vi "main.vi"() -> ()   [LabVIEW 2012]
uses:
  SensorSettingCtl.ctl
  SensorTypes.ctl
  states.ctl
  globalVariables.vi
panel:
  in  "cancel button":bool
  out "TestLED":bool
  in  "Path for measuring results":path
  in  "Configuration of sensors":T1[](array[typedef])=[{"Sensor type"=enum."please select sensor", "Sensor on"=FALSE, "VISA resource name"="", "current transfer ratio"=0.0, "DMM Channel"="", "NPLC"=2, "Range"=enum."Maximum"}, {"Sensor type"=enum."ITL 900 (Analogue)", "Sensor on"=TRUE, "VISA resource name"="", "current transfer ratio"=0.0, "DMM Channel"="", "NPLC"=2, "Range"=enum."Maximum"}, {"Sensor type"=enum."CAB 300-C SP3 (CAN)", "Sensor on"=TRUE, "VISA resource name"="", "current transfer ratio"=0.0, "DMM Channel"="", "NPLC"=2, "Range"=enum."Maximum"}] {"NPLC" items=[".02", ".2", "1", "2", "10", "20", "100", "200", "Minimum", "Maximum"]}
  in  "start Button":bool
  out "Error Flag":bool
  # "Measurement of Current Sensors from LEM"
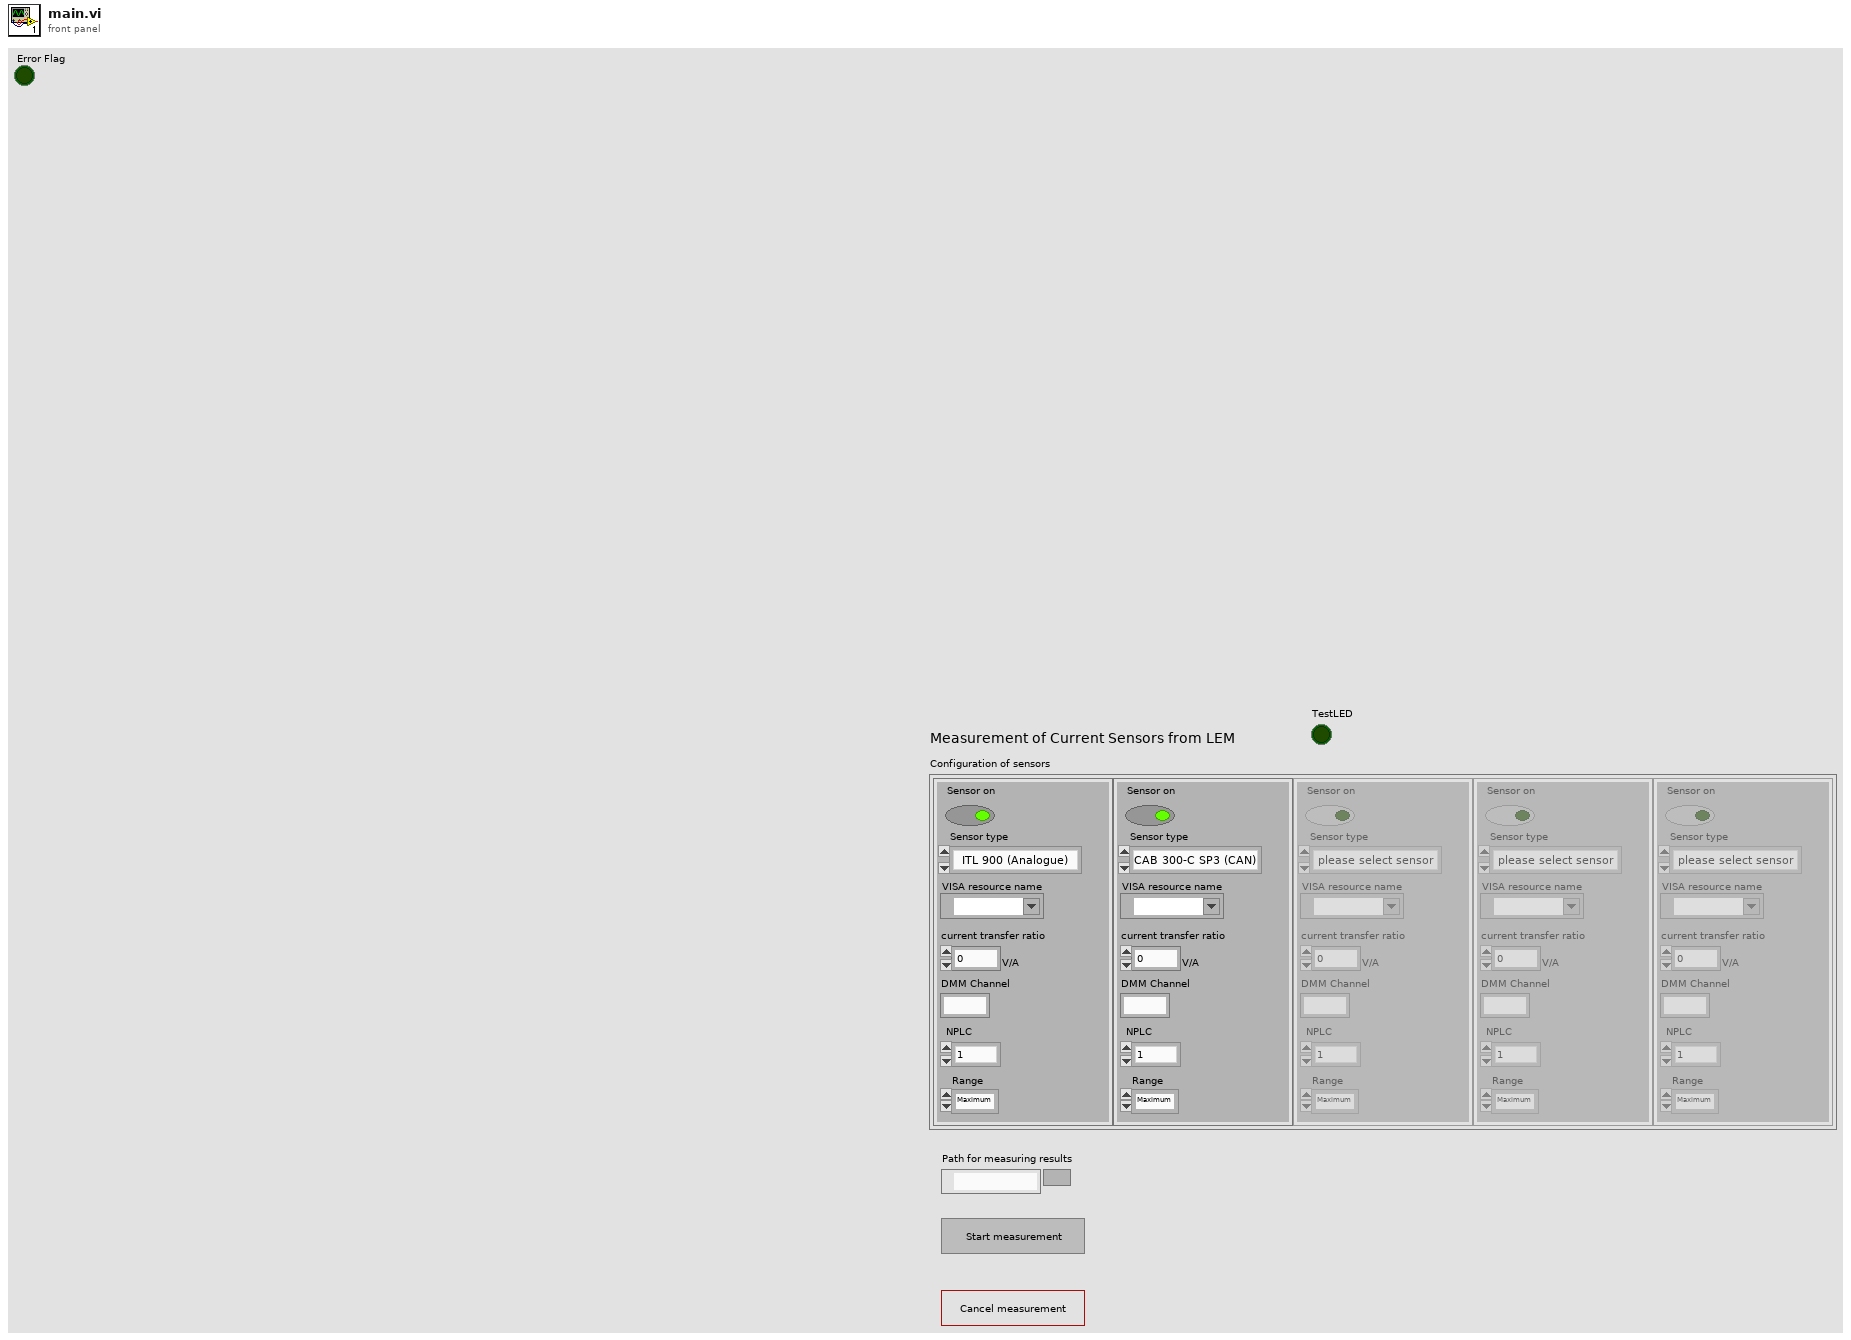
[diagram p1: front panel]
types:
  T1 = typedef "SensorSettingCtl.ctl" = cluster{"Sensor type":T2, "Sensor on":bool, "VISA resource name":refnum<visa-resource-name>, "current transfer ratio":dbl[unit], "DMM Channel":string, "NPLC":u16, "Range":enum16{"100 mV", "1 V", "10 V", "100 V", "300 V", "Minimum", "Maximum"}}
  T2 = typedef "SensorTypes.ctl" = enum16{"please select sensor", "ITL 900 (Analogue)", "CAB 300-C SP3 (CAN)", "xyz TODO (LIN)", "xyz TODO (Analogue)", "xyz TODO (CAN)"}
  T3 = typedef "states.ctl" = enum16{"init", "wait for user confirm", "start sensors", "measure", "terminate"}
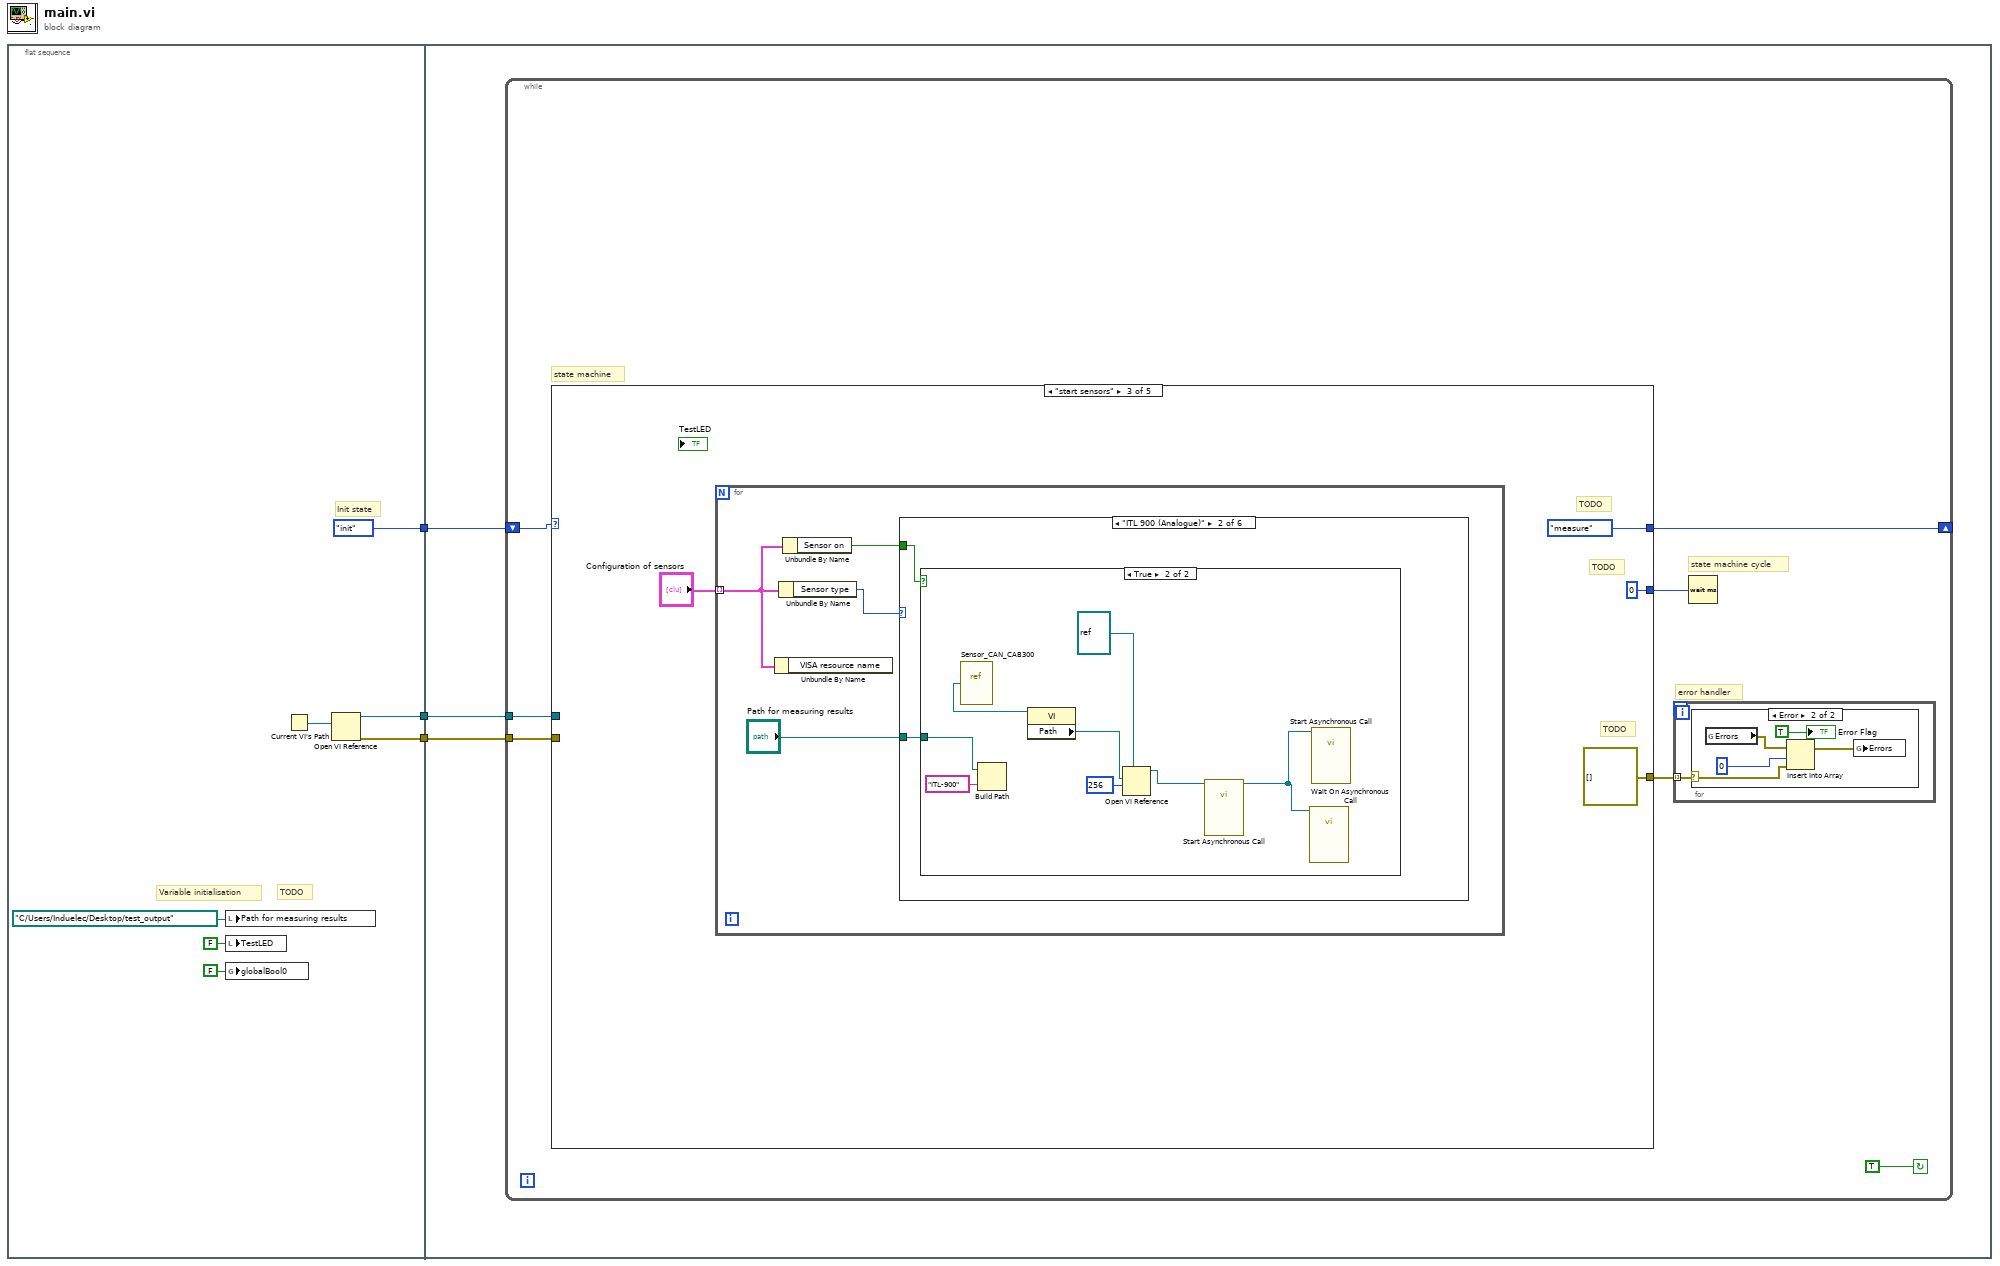
[diagram p0: block diagram]
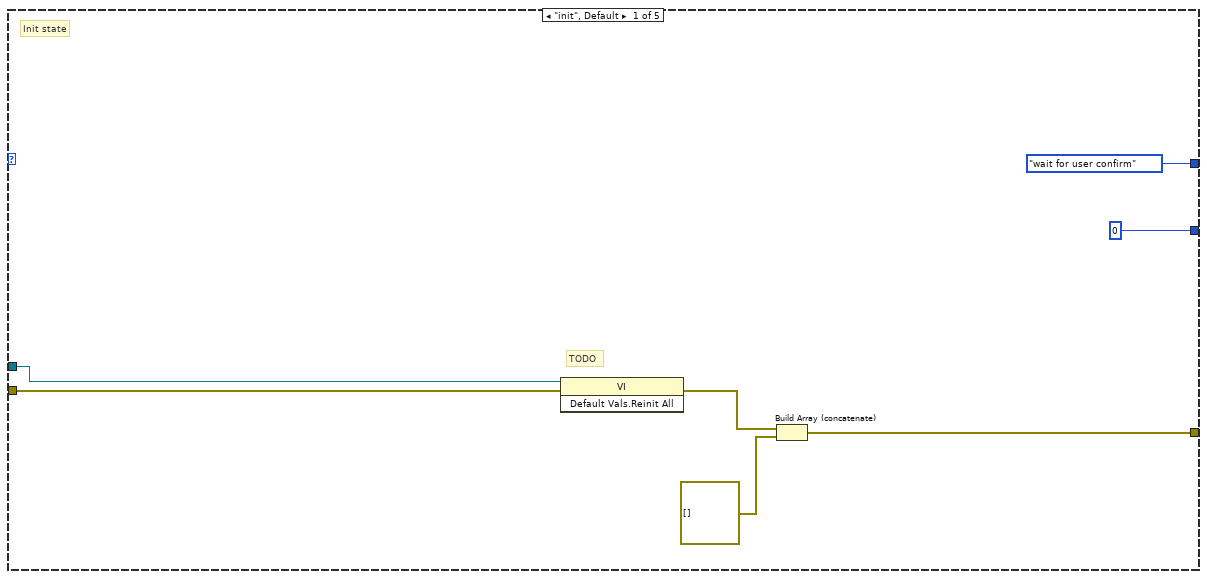
[diagram p3: hidden frame]
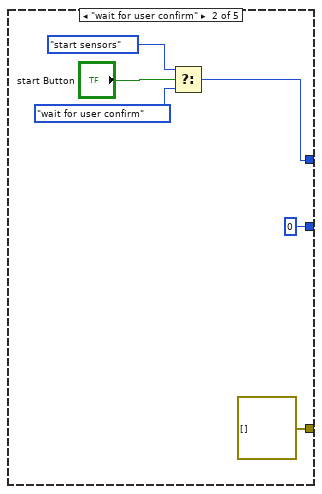
[diagram p4: hidden frame]
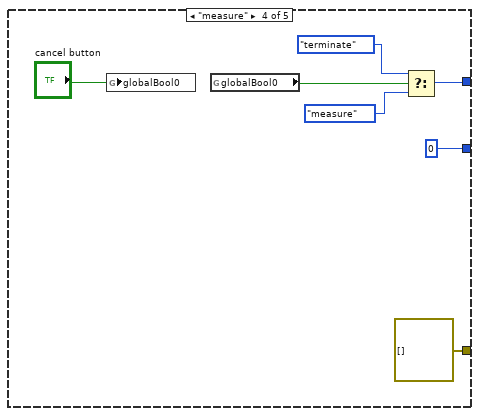
[diagram p11: hidden frame]
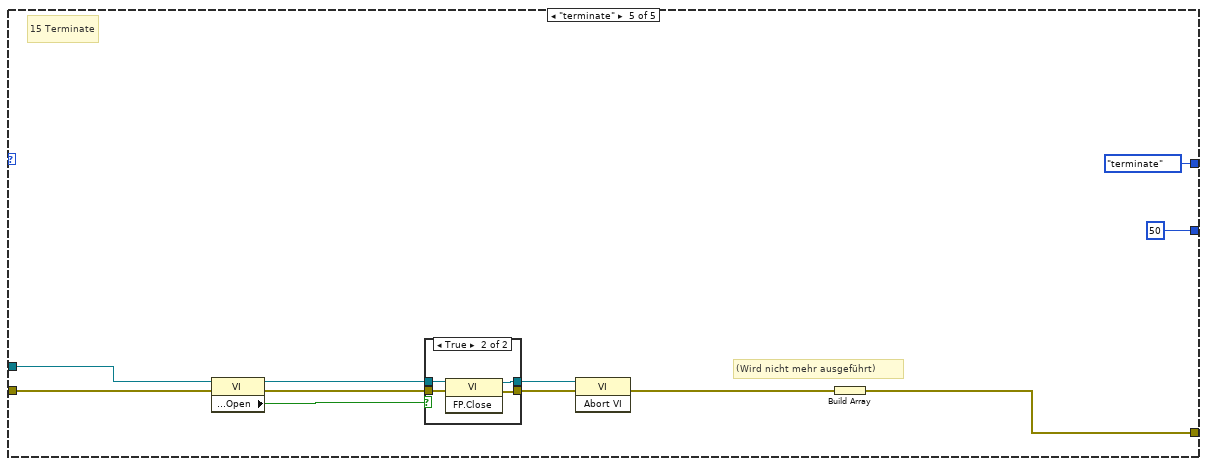
[diagram p12: hidden frame]
diagram:
  n1 = flat-sequence {
    tunnel: [states."init" ("States IEEE-488")] -> w3
    tunnel: [w10] -> w2
    tunnel: [w9] -> w1
    tunnel: w3 -> [w11]
    tunnel: w2 -> [w13]
    tunnel: w1 -> [w12]
    frame #0 {
      # "TODO"
      # "Variable initialisation"
      # "Init state"
      n2 = local write "Path for measuring results"(path "C:/Users/Induelec/Desktop/test_output" ("Path for measuring results")) -> ()
      n3 = local write "TestLED"(FALSE ("both Tests are running")) -> ()
      n4 = global write "globalVariables.vi" "globalBool0"(FALSE ("globalBool0")) -> ()
      n5 = Current VI's Path() -> (path=w8:path)
      n6 = Open VI Reference(vi path=w8) -> (vi reference=w10:refnum<vi>, error out=w9:errorcluster)  [unwired: 2 in, 3 out]
    }
    frame #1 {
      n7 = while {
        tunnel: w13 -> [w18]
        tunnel: w12 -> [w17]
        shift-right: [w14] -> _
        shift-left: w11 -> [w15]
        stop <- TRUE continue-if-true
        # "state machine"
        # "error handler"
        # "state machine cycle"
        n8 = case shown="\"start sensors\"" w15 {
          tunnel: [u32 0 ("milliseconds to wait") u32 0 ("milliseconds to wait") u32 0 ("milliseconds to wait") u32 0 ("milliseconds to wait") u32 50 ("milliseconds to wait")] -> w19
          tunnel: w18 -> [w30 _ _ _ w68]
          tunnel: w17 -> [w31 _ _ _ w69]
          tunnel: [w32 errorcluster[] [] errorcluster[] [] errorcluster[] [] w73] -> w16
          tunnel: [states."wait for user confirm" ("States IEEE-488") w36 states."measure" ("States IEEE-488") w61 states."terminate" ("f")] -> w14
          frame "init", Default {
            # "Init state"
            # "TODO"
            n9 = invoke class="VI" method="Default Vals.Reinit All"(reference=w30, error in=w31) -> (error out=w29:errorcluster)  [unwired: 1 in, 2 out]
            n10 = Build Array (concatenate)(w29, errorcluster[] [] ("array")) -> (w32:errorcluster[])
          }
          frame "wait for user confirm" {
            n11 = Select(t=states."start sensors" ("States IEEE-488"), s="start Button", f=states."wait for user confirm" ("States IEEE-488")) -> (s? t:f=w36:T3)
          }
          frame "start sensors" {
            # "TODO"
            # "TODO"
            # "TODO"
            n12 = for {
              tunnel: "Configuration of sensors" -> [w46] mode=indexing
              n13 = Unbundle By Name(w46) -> ()  [unwired: 1 out]
              n14 = Unbundle By Name(w46) -> ("Sensor type"=w47:T2)
              n15 = Unbundle By Name(w46) -> ("Sensor on"=w45:bool)
              n16 = case shown="\"ITL 900 (Analogue)\"" w47 {
                tunnel: w45 -> [_ w49 _ _ _ _]
                tunnel: "Path for measuring results" -> [_ w48 _ _ _ _]
                frame "please select sensor", Default {
                }
                frame "ITL 900 (Analogue)" {
                  n17 = case shown="True" w49 {
                    tunnel: w48 -> [_ w51]
                    frame False {
                    }
                    frame True {
                      n18 = vi-ref "Sensor_CAN_CAB300.vi"() -> (w57:refnum<vi>)
                      n19 = Build Path(base path=w51, name or relative path="ITL-900") -> ()  [unwired: 1 out]
                      n20 = property class="VI"(reference=w57) -> ("Path"=w56:path)  [unwired: 1 in, 2 out]
                      n21 = Open VI Reference(type specifier VI Refnum (for type only)=refnum<vi> refnum, vi path=w56, options=256) -> (vi reference=w54:refnum<vi>)  [unwired: 3 in, 1 out]
                      n22 = call-by-ref "Start Asynchronous Call"(reference=w54) -> (reference out=w52:refnum<vi>)  [unwired: 13 in, 1 out]
                      n23 = call-by-ref "Wait On Asynchronous Call"(reference=w52) -> ()  [unwired: 13 in, 2 out]
                      n24 = call-by-ref "Start Asynchronous Call"(reference=w52) -> ()  [unwired: 13 in, 2 out]
                    }
                  }
                }
                frame "CAB 300-C SP3 (CAN)" {
                }
                frame "xyz TODO (LIN)" {
                }
                frame "xyz TODO (Analogue)" {
                }
                frame "xyz TODO (CAN)" {
                }
              }
            }
          }
          frame "measure" {
            n25 = global write "globalVariables.vi" "globalBool0"("cancel button") -> ()
            n26 = global read "globalVariables.vi" "globalBool0"() -> (w63:bool)
            n27 = Select(t=states."terminate" ("States IEEE-488"), s=w63, f=states."measure") -> (s? t:f=w61:T3)
          }
          frame "terminate" {
            # "(Wird nicht mehr ausgeführt)"
            # "15 Terminate"
            n28 = property class="VI"(reference=w68, error in=w69) -> (reference out=w71:refnum<vi>, error out=w70:errorcluster, "Front Panel.Open"=w72:bool)
            n29 = case shown="True" w72 {
              tunnel: w71 -> [w77 w81]
              tunnel: [w77 w80] -> w67
              tunnel: w70 -> [w76 w79]
              tunnel: [w76 w78] -> w66
              frame False {
              }
              frame True {
                n30 = invoke class="VI" method="FP.Close"(reference=w81, error in=w79) -> (reference out=w80:refnum<vi>, error out=w78:errorcluster)  [unwired: 1 in, 1 out]
              }
            }
            n31 = invoke class="VI" method="Abort VI"(reference=w67, error in=w66) -> (error out=w74:errorcluster)  [unwired: 1 in, 2 out]
            n32 = Build Array(w74) -> (w73:errorcluster[])
          }
        }
        n33 = for {
          tunnel: w16 -> [w21] mode=indexing
          n34 = case shown="Error" w21 {
            selector: w21 -> [_ w25]
            frame No Error {
            }
            frame Error {
              n35 = global read "globalVariables.vi" "Errors"() -> (w23:errorcluster[])
              n36 = Insert Into Array(array=w23, index=0, new element=w25) -> (w22:errorcluster[])
              n37 = global write "globalVariables.vi" "Errors"(w22) -> ()
              "Error Flag" <- TRUE ("Error Flag")
            }
          }
        }
        n38 = Wait (ms)(milliseconds to wait=w19) -> ()  [unwired: 1 out]
      }
    }
  }
